vi "GetCalibrData.vi"(8 "error in (no error)":errorcluster, 10 "Mode":T1, 11 "Refnum in":refnum<visa-resource-name>) -> (0 "error out":errorcluster, 1 "INT":i32[][](array[numeric]))   [LabVIEW 2020]
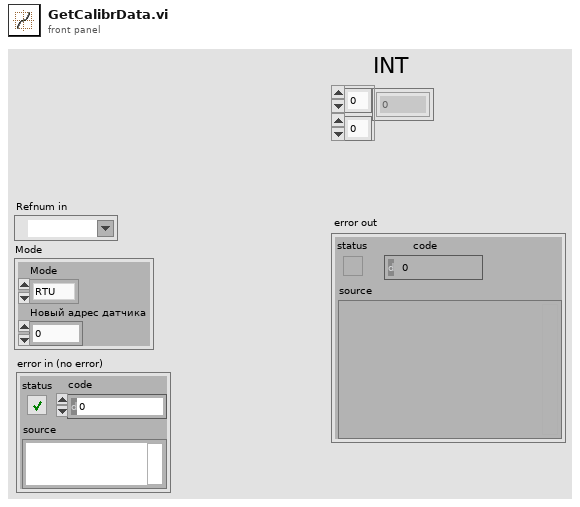
[diagram p1: front panel]
types:
  T1 = cluster{"Mode":enum16{"RTU", "ASCII"}, "Новый адрес датчика":u16}
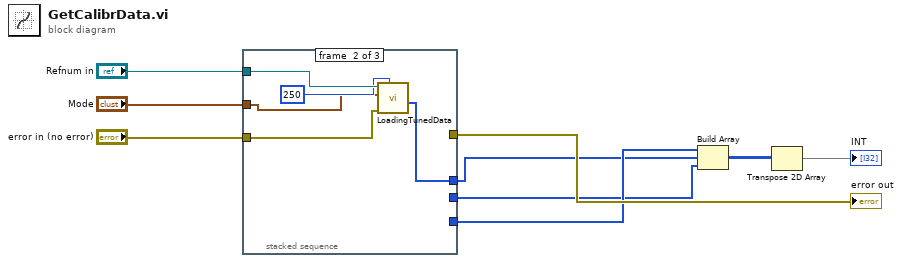
[diagram p0: block diagram]
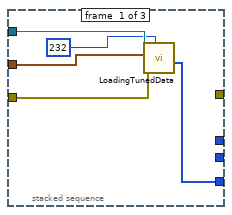
[diagram p2: hidden frame]
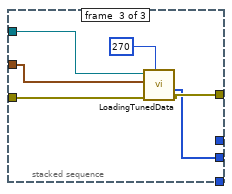
[diagram p3: hidden frame]
diagram:
  n1 = stacked-sequence {
    tunnel: "Refnum in" -> [w14 w19 w25]
    tunnel: "Mode" -> [w11 w16 w23]
    tunnel: "error in (no error)" -> [w13 w18 w24]
    tunnel: [_ _ w21] -> w6
    tunnel: [w10 _ _] -> w5
    tunnel: [_ w15 _] -> w4
    tunnel: [_ _ w20] -> w3
    frame #0 {
      n2 = call "LoadingTunedData.vi"("Refnum in"=w14, "Mode"=w11, "error in (no error)"=w13, "StartAddr"=232) -> ("INT"=w10:i32[])  [unwired: 5 in, 1 out]
    }
    frame #1 {
      n3 = call "LoadingTunedData.vi"("Refnum in"=w19, "Mode"=w16, "error in (no error)"=w18, "StartAddr"=250) -> ("INT"=w15:i32[])  [unwired: 5 in, 1 out]
    }
    frame #2 {
      n4 = call "LoadingTunedData.vi"("Refnum in"=w25, "Mode"=w23, "error in (no error)"=w24, "StartAddr"=270) -> ("INT"=w20:i32[], "error out"=w21:errorcluster)  [unwired: 5 in]
    }
  }
  "error out" <- w6
  n5 = Build Array(w5, w4, w3) -> (w1:i32[][])
  n6 = Transpose 2D Array(2D array=w1) -> (transposed array=→"INT":i32[][])
